vi "HT3_Finish.vi"(4 "Input 1 Rate":i32, 5 "FileHeaderPos":T1, 6 "Input 0 Rate":i32, 7 "Stop Reason":enum16{"timeover", "manual", "overflow"}(ring), 8 "error in":errorcluster, 9 "Num Records":i64, 10 "Stop After (ms)":i32, 11 "refnum in":refnum<file>) -> (0 "error out":errorcluster)   [LabVIEW 2013]
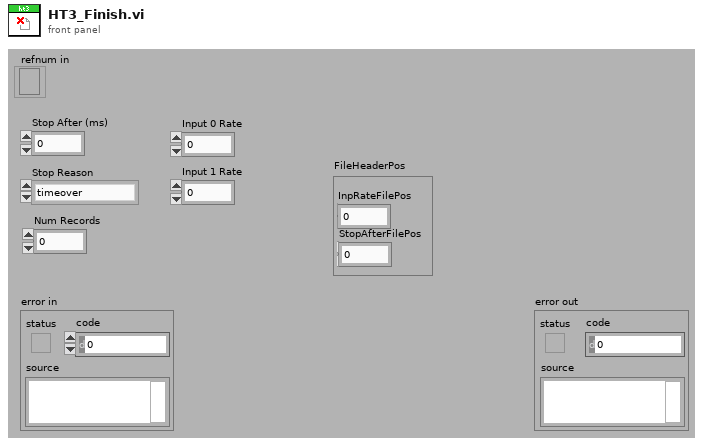
[diagram p1: front panel]
types:
  T1 = cluster{"InpRateFilePos":i64, "StopAfterFilePos":i64}
  T2 = enum16{"big-endian, network order", "native, host order", "little-endian"}
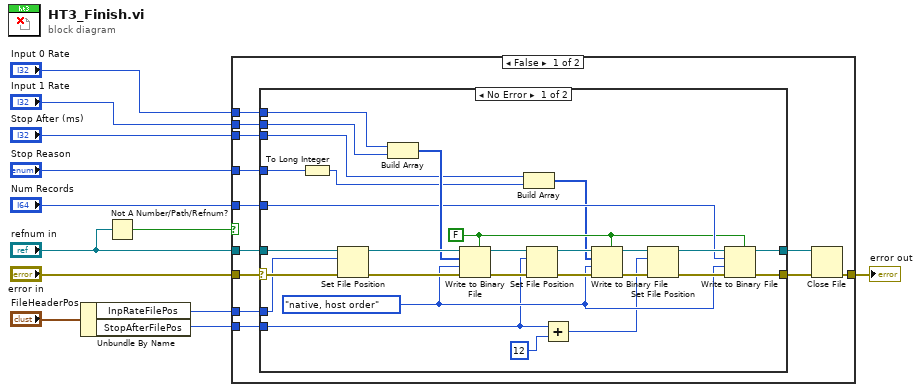
[diagram p0: block diagram]
diagram:
  n1 = Unbundle By Name("FileHeaderPos") -> ("InpRateFilePos"=w2:i64, "StopAfterFilePos"=w1:i64)
  n2 = Not A Number/Path/Refnum?(number/path/refnum="refnum in") -> (NaN/Path/Refnum?=w7:bool)
  n3 = case shown="False" w7 {
    tunnel: "error in" -> [w24 w55]
    tunnel: "refnum in" -> [w23 _]
    tunnel: [w22 w55] -> w11
    tunnel: "Stop Reason" -> [w19 _]
    tunnel: "Num Records" -> [w18 _]
    tunnel: "Stop After (ms)" -> [w17 _]
    tunnel: "Input 1 Rate" -> [w16 _]
    tunnel: "Input 0 Rate" -> [w15 _]
    tunnel: w2 -> [w14 _]
    tunnel: w1 -> [w13 _]
    frame False {
      n4 = case shown="No Error" w24 {
        selector: w24 -> [w52 w53]
        tunnel: w23 -> [w51 w54]
        tunnel: [w37 w53] -> w21
        tunnel: [w32 w54] -> w20
        tunnel: w19 -> [w48 _]
        tunnel: w18 -> [w31 _]
        tunnel: w17 -> [w43 _]
        tunnel: w16 -> [w46 _]
        tunnel: w15 -> [w45 _]
        tunnel: w14 -> [w44 _]
        tunnel: w13 -> [w27 _]
        frame No Error {
          w30 = T2."native, host order" ("byte order (0:big-endian, network order)")
          w29 = FALSE ("prepend array or string size? (T)")
          n5 = To Long Integer(number=w48) -> (32bit integer=w42:i32)
          n6 = Set File Position(offset (in bytes) (0)=w44, refnum=w51, error in=w52) -> (refnum out=w49:refnum<file>, error out=w50:errorcluster)  [unwired: 1 out]
          n7 = Build Array(w45, w46) -> (w47:i32[])
          n8 = Write to Binary File(file (use dialog)=w49, data=w47, error in=w50, 5:w29, 9:w30) -> (refnum out=w36:refnum<file>, error out=w41:errorcluster)  [unwired: 2 out]
          n9 = Build Array(w43, w42) -> (w28:i32[])
          n10 = Set File Position(offset (in bytes) (0)=w27, refnum=w36, error in=w41) -> (refnum out=w35:refnum<file>, error out=w40:errorcluster)  [unwired: 1 in]
          n11 = Add(x=w27, y=i64 12) -> (x+y=w25:i64)
          n12 = Write to Binary File(file (use dialog)=w35, data=w28, error in=w40, 5:w29, 9:w30) -> (refnum out=w34:refnum<file>, error out=w39:errorcluster)  [unwired: 2 out]
          n13 = Set File Position(offset (in bytes) (0)=w25, refnum=w34, error in=w39) -> (refnum out=w33:refnum<file>, error out=w38:errorcluster)  [unwired: 1 out]
          n14 = Write to Binary File(file (use dialog)=w33, data=w31, error in=w38, 5:w29, 9:w30) -> (refnum out=w32:refnum<file>, error out=w37:errorcluster)  [unwired: 2 out]
        }
        frame Error {
        }
      }
      n15 = Close File(refnum=w20, error in=w21) -> (error out=w22:errorcluster)  [unwired: 1 out]
    }
    frame True {
    }
  }
  "error out" <- w11
